vi "Testschedulev2.vi"() -> ()   [LabVIEW 2014]
uses:
  <vilib>/Utility/miscctls.llb/LVRowAndColumnTypeDef.ctl
  <vilib>/Utility/miscctls.llb/LVBoundsTypeDef.ctl
  <vilib>/event_ctls.llb/eventvkey.ctl
  <vilib>/platform/TimedLoop/XDataNode/XDataNode.xnode
  <vilib>/Platform/TimedLoop/XDataNode/timing_clust.ctl
  <vilib>/Platform/TimedLoop/XDataNode/XDNodeRunTimeDep.lvlib
  <vilib>/Platform/TimedLoop/XDataNode/wakeup.ctl
  <vilib>/Platform/TimedLoop/XDataNode/nitl_modes.ctl
panel:
  in  "Loop Number":i32
  in  "Test Flow rate g/s":i32
  in  "Test Type":u16(ring) items=["CO Lightoff", "HC Lightoff", "NO Lightoff", "OSC", "Ageing", "Leak"]
  out "Test Start":bool
  out "Loop Number":i32
  in  "Test Ready":bool
  in  "% Complete":i32(slide) scale=0.0..100.0
  in  "Time to Complete":dbl
  in  "Main TC":i32
  in  "Fan Speed V":i32
  in  "Inlet Temperature (°C)":i32
  in  "Cycle Name":string
  in  "Cycle Length":i32
  in  "Test Number":i32
  in  "Test Type Items":string[](array[string])=["CO Lightoff", "HC Lightoff", "NO Lightoff", "OSC", "Ageing", "Leak"]
  in  "TC Items":string[](array[string])=["TC1", "TC2", "TC3", "TC4", "TC5", "TC6"]
  in  "Recipe Items":string[](array[string])=["LeanspikeV1.eyes", "RAT060619Z1.eyes", "RAT181206KTM617.eyes", "RAT181217RichSpike.eyes", "RAT190207KTM934.eyes", "RAT190319KTM943Tune.eyes", "RAT190401.eyes", "RAT190405.eyes", "RAT190405e.eyes", "RAT190405f.eyes", "RAT190405g.eyes", "RAT190405h.eyes", "RAT190405i.eyes", "RAT190405j.eyes", "RAT190405k.eyes", "RAT190405L.eyes", "RAT190405M.eyes", "RAT190405N.eyes", "RAT190405O.eyes", "RAT190405P.eyes", "RAT190405Q.eyes", "RAT190405R.eyes", "RAT190405S.eyes", "RAT190405T.eyes", "RAT190405U.eyes", "RAT190405V.eyes", "RAT190405W.eyes", "RAT190405Y.eyes", "RAT190405Y2.eyes", "RAT190405Z.eyes", "RATAMP.eyes", "Richspike.eyes", "ZERO.eyes"]
  in  "Test Size":i32=2
  in  "Selection Finished":bool
  in  "Duration":i32=10 min=0
  in  "Recipe":u16(ring)=32 items=["LeanspikeV1.eyes", "RAT060619Z1.eyes", "RAT181206KTM617.eyes", "RAT181217RichSpike.eyes", "RAT190207KTM934.eyes", "RAT190319KTM943Tune.eyes", "RAT190401.eyes", "RAT190405.eyes", "RAT190405e.eyes", "RAT190405f.eyes", "RAT190405g.eyes", "RAT190405h.eyes", "RAT190405i.eyes", "RAT190405j.eyes", "RAT190405k.eyes", "RAT190405L.eyes", "RAT190405M.eyes", "RAT190405N.eyes", "RAT190405O.eyes", "RAT190405P.eyes", "RAT190405Q.eyes", "RAT190405R.eyes", "RAT190405S.eyes", "RAT190405T.eyes", "RAT190405U.eyes", "RAT190405V.eyes", "RAT190405W.eyes", "RAT190405Y.eyes", "RAT190405Y2.eyes", "RAT190405Z.eyes", "RATAMP.eyes", "Richspike.eyes", "ZERO.eyes"]
  in  "TC":u16(ring) items=["TC1", "TC2", "TC3", "TC4", "TC5", "TC6"]
  in  "Temperature":i32=10 min=0
  in  "Flow":i32=10 min=0
  out "Test Schedule":string[][](table)=[["OSC", "0", "ZERO.eyes", "0", "0", "TC1"], ["OSC", "0", "ZERO.eyes", "0", "0", "TC1"]]
  in  "Update Recipe List":bool
  out "Listbox":i32(listbox)
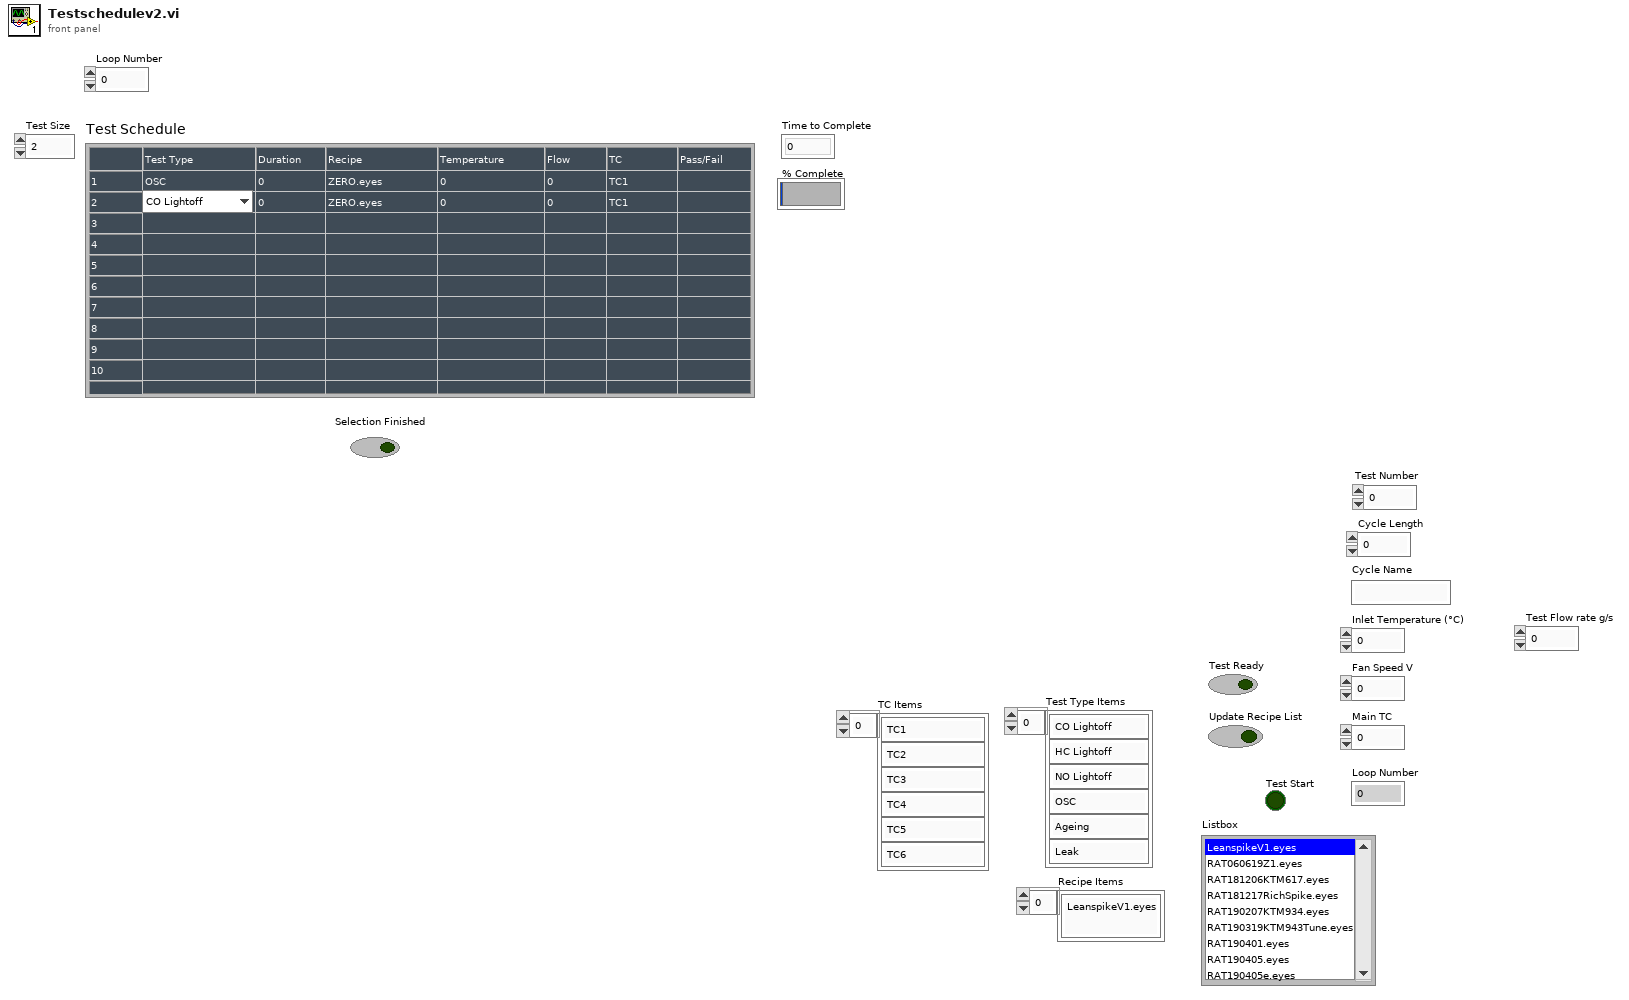
[diagram p1: front panel]
types:
  T1 = cluster{"Test Type":u16, "Duration":i32, "Recipe":u16, "Temperature":i32, "Flow":i32, "TC":u16}
  T2 = typedef "LVRowAndColumnTypeDef.ctl" = cluster{"Row":i32, "Column":i32}
  T3 = cluster{"Test Type":u16, "Duration":i32, "Recipe":u16, "Temperature":i32, "Flow":i32, "TC":u16}[]
  T4 = cluster{i32[], i32[], "Recipe":string[], i32[], i32[], i32[], bool[]}
  T5 = typedef "LVBoundsTypeDef.ctl" = cluster{"Width":u32, "Height":u32}
  T6 = typedef "eventvkey.ctl" = enum16{"ASCII", "Enter", "Return", "Shift", "Ctrl", "Alt", "Cmd", "Opt", "Caps", "NumLock", "Clear", "Break", "Up", "Down", "Left", "Right", "Insert", "Delete", "Home", "End", "PageUp", "PageDown", "Escape", "Help", "Pause", "ScrollLock", "F1", "F2", "F3", "F4", "F5", "F6", "F7", "F8", "F9", "F10", "F11", "F12", "F13", "F14", "F15", "F16", "F17", "F18", "F19", "F20", "F21", "F22", "F23", "F24", "Play", "VolumeUp", "VolumeDown", "Mute", "Two Byte Char"}
  T7 = typedef "LVPoint32TypeDef.ctl" = cluster{"Horizontal":i32, "Vertical":i32}
  T8 = typedef "LVPositionTypeDef.ctl" = cluster{"Left":i32, "Top":i32}
  T9 = cluster{"Shift":bool, "Ctrl":bool, "Alt":bool, "Cmd":bool, "Opt":bool}
  T10 = cluster{"Array":string[], "Array 2":string[], "Array 3":string[], "Array 4":string[], "Array 5":string[], "Array 6":string[]}
  T11 = cluster{i32[], i32[], "Array 3":string[], i32[], i32[], i32[], bool[]}
  T12 = cluster{i32, i32, "Combo Box":string, i32, i32, "index":i32}
  T13 = typedef "XDNodeRunTimeDep.lvlib/timing_clust.ctl" = cluster{"Expected End [f-1]":u64, "Actual End [f-1]":u64, "Finished Late? [f-1]":bool, "Expected End [i-1]":u64, "Actual End [i-1]":u64, "Finished Late? [i-1]":bool, "Expected Start [i]":u64, "Actual Start [i]":u64, "Expected Start [f]":u64, "Actual Start [f]":u64, "Source Name":string, "Structure Name":string, "Period":i64, "Deadline":i64, "Offset":i64, "Start":i64, "Priority":i32, "Timeout":i32, "Mode":T14, "Wakeup Reason":T15, "Error":errorcluster, "Source Type":string, "Secondary Source Type":string, "Global End Time":u64, "Global Start Time":u64, "Frame Duration":u64, "Iteration Duration":u64, "Assigned CPU":i32, "I/O Scan Engine Mode":u32}
  T14 = typedef "XDNodeRunTimeDep.lvlib/nitl_modes.ctl" = enum32{"No Change", "Process missed periods, maintain original phase", "Discard missed periods, maintain original phase", "Process missed periods, ignore original phase", "Discard missed periods, ignore original phase"}
  T15 = typedef "XDNodeRunTimeDep.lvlib/wakeup.ctl" = enum32{"Normal", "Aborted", "Asynchronous wakeup", "Timing source error", "Timed loop error", "Timeout"}
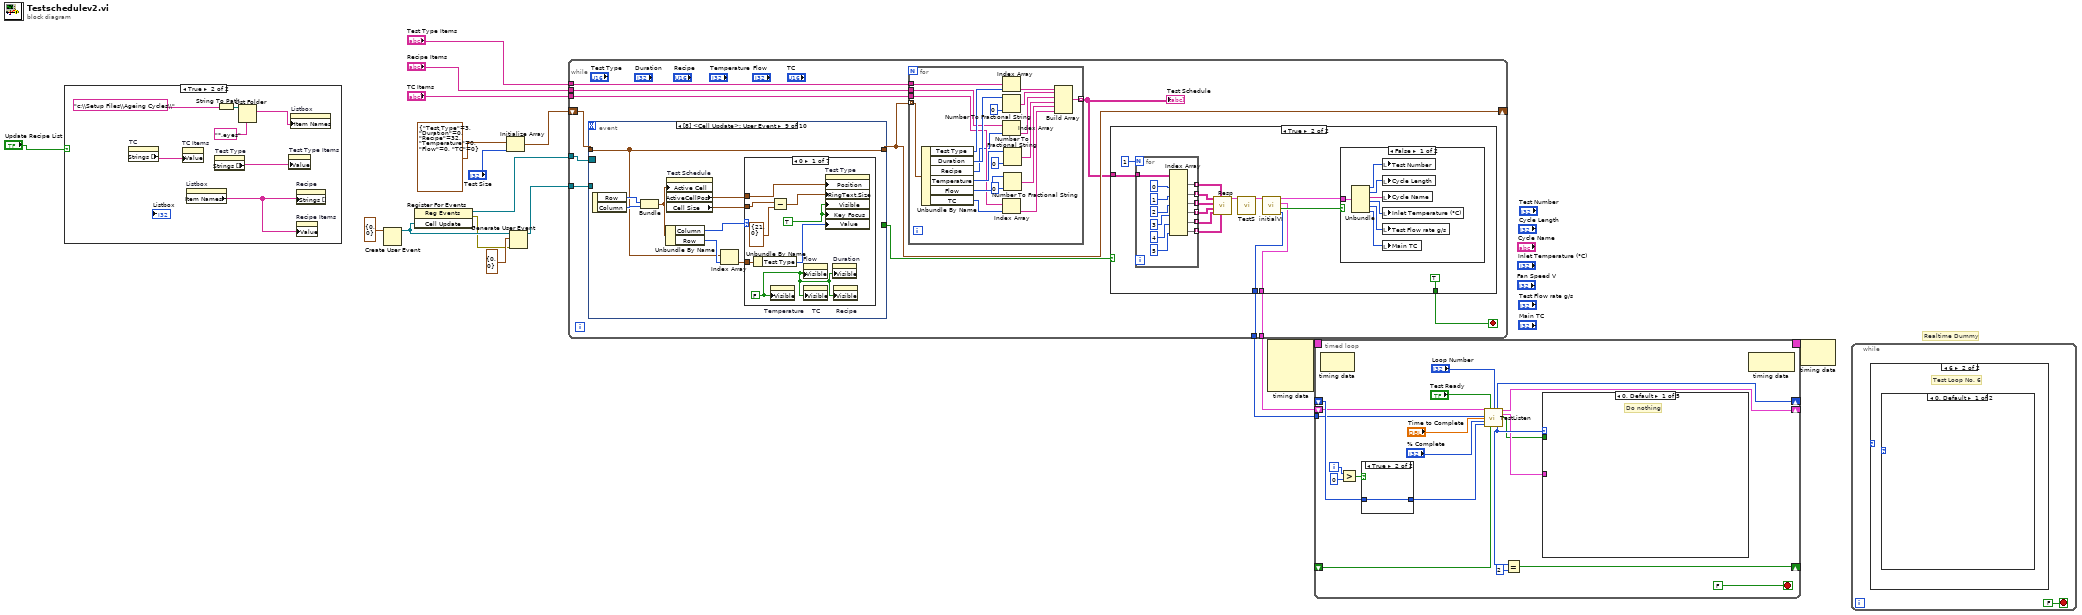
[diagram p0: block diagram]
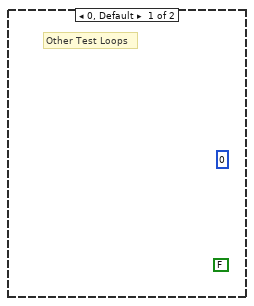
[diagram p2: hidden frame]
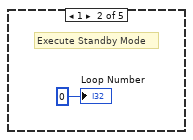
[diagram p4: hidden frame]
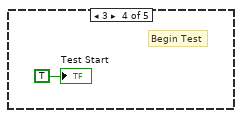
[diagram p6: hidden frame]
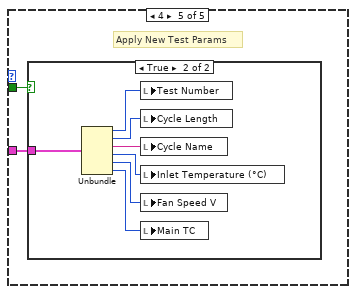
[diagram p7: hidden frame]
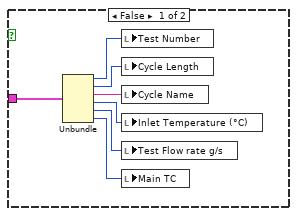
[diagram p8: hidden frame]
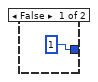
[diagram p9: hidden frame]
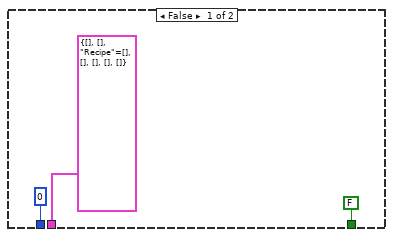
[diagram p10: hidden frame]
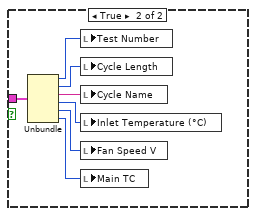
[diagram p11: hidden frame]
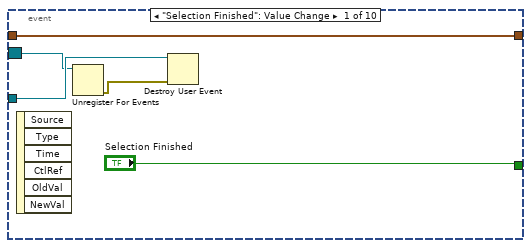
[diagram p12: hidden frame]
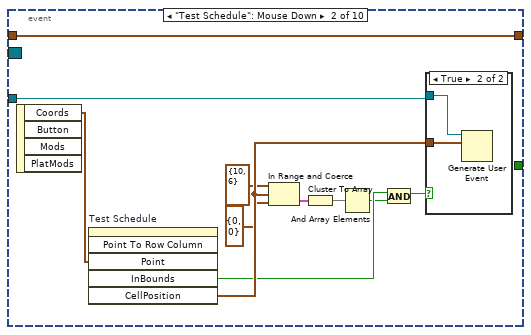
[diagram p13: hidden frame]
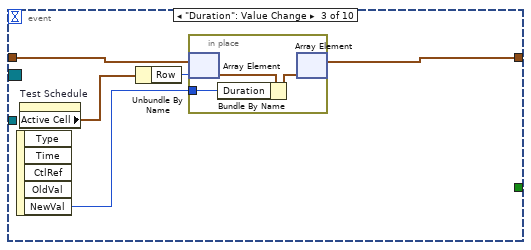
[diagram p15: hidden frame]
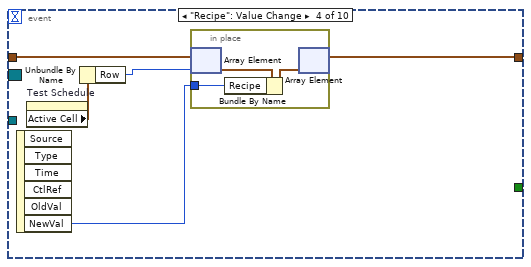
[diagram p16: hidden frame]
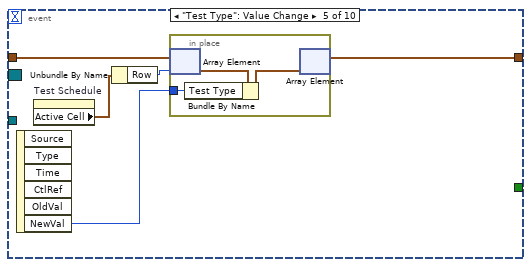
[diagram p17: hidden frame]
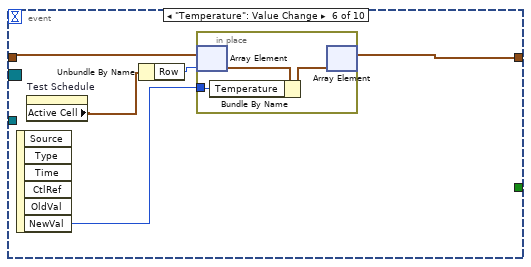
[diagram p18: hidden frame]
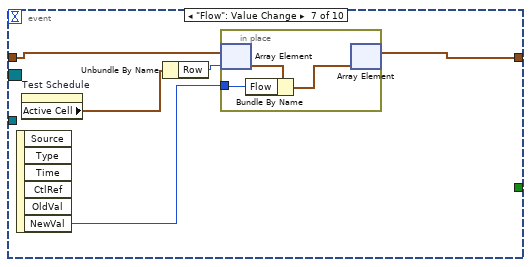
[diagram p19: hidden frame]
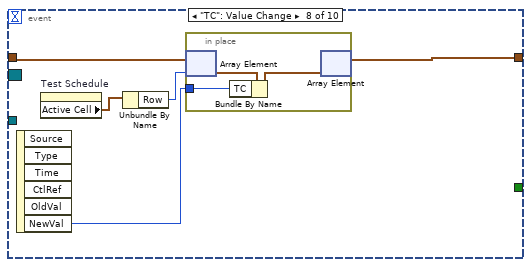
[diagram p20: hidden frame]
diagram:
  # "Realtime Dummy"
  n1 = case shown="True" "Update Recipe List" {
    frame False {
    }
    frame True {
      n2 = property on="TC" class="Ring (strict)"() -> ("Strings []"=w20:string[])  [unwired: 2 in, 2 out]
      n3 = property on="TC Items" class="Arr (strict)"("Value"=w20) -> ()  [unwired: 2 in, 2 out]
      n4 = property on="Listbox" class="LstBox (strict)"() -> ("Item Names"=w19:string[])  [unwired: 2 in, 2 out]
      n5 = property on="Test Type" class="Ring (strict)"() -> ("Strings []"=w18:string[])  [unwired: 2 in, 2 out]
      n6 = String To Path(string="c:\\Setup Files\\Ageing Cycles\\") -> (path=w24:path)
      n7 = List Folder(path=w24, pattern="*.eyes") -> (filenames=w21:string[])  [unwired: 2 in, 3 out]
      n8 = property on="Test Type Items" class="Arr (strict)"("Value"=w18) -> ()  [unwired: 2 in, 2 out]
      n9 = property on="Listbox" class="LstBox (strict)"("Item Names"=w21) -> ()  [unwired: 2 in, 2 out]
      n10 = property on="Recipe" class="Ring (strict)"("Strings []"=w19) -> ()  [unwired: 2 in, 2 out]
      n11 = property on="Recipe Items" class="Arr (strict)"("Value"=w19) -> ()  [unwired: 2 in, 2 out]
    }
  }
  n12 = Create User Event(user event datatype=T2 {"Row"=0, "Column"=0} ("Cell Update")) -> (user event=w11:refnum<user-event>)  [unwired: 1 in, 1 out]
  n13 = register-events(w11) -> (reference out=w13:refnum<event-registration>, error out=w9:errorcluster)  [unwired: 2 in]
  n14 = Initialize Array(T1 {"Test Type"=3, "Duration"=0, "Recipe"=32, "Temperature"=0, "Flow"=0, "TC"=0} ("Dilution Product Selection"), "Test Size") -> (w15:T3)
  n15 = Generate User Event(user event=w11, event data cluster=T2 {"Row"=0, "Column"=0} ("event data"), error in=w9) -> (user event out=w8:refnum<user-event>)  [unwired: 1 in, 1 out]
  n16 = while {
    shift-right: [w34] -> _
    shift-left: w15 -> [w36]
    tunnel: w13 -> [w35]
    tunnel: w8 -> [w33]
    tunnel: "Test Type Items" -> [w32]
    tunnel: "Recipe Items" -> [w31]
    tunnel: "TC Items" -> [w30]
    tunnel: [w28] -> w2
    tunnel: [w27] -> w1
    stop <- w26 stop-if-true
    n17 = event shown="[8] <Cell Update>: User Event" {
      selector: w35 -> [w104 _ _ _ _ _ _ _ _ _]
      dyn-events: _ -> [_ _ _ _ _ _ _ _ _ _]
      timeout: _ -> [_ _ _ _ _ _ _ _ _ _]
      tunnel: w36 -> [w106 w109 w124 w131 w140 w145 w154 w162 w168 w241]
      tunnel: [w106 w109 w122 w128 w138 w144 w152 w160 w168 w241] -> w34
      tunnel: w33 -> [w105 w108 _ _ _ _ _ _ _ w219]
      tunnel: ["Selection Finished" _ _ _ _ _ _ _ _ _] -> w25
      event "Selection Finished": Value Change {
        n18 = event-data() -> ()  [unwired: 1 in, 6 out]
        n19 = Destroy User Event(user event=w105) -> (error out=w103:errorcluster)  [unwired: 1 in]
        n20 = Unregister For Events(event registration refnum=w104, error in=w103) -> ()  [unwired: 1 out]
      }
      event "Test Schedule": Mouse Down {
        n21 = event-data() -> ("Coords"=w107:T7)  [unwired: 1 in, 3 out]
        n22 = invoke on="Test Schedule" class="Tbl (strict)" method="Point To Row Column"("Point"=w107) -> ("InBounds"=w113:bool, "CellPosition"=w117:T2)  [unwired: 5 in, 4 out]
        n23 = In Range and Coerce(upper limit=T2 {"Row"=10, "Column"=6}, x=w117, lower limit=T2 {"Row"=0, "Column"=0}) -> (In Range?=w114:cluster{"Row":bool, "Column":bool})  [unwired: 1 out]
        n24 = Cluster To Array(cluster=w114) -> (array=w111:bool[])
        n25 = And Array Elements(Boolean array=w111) -> (logical AND=w110:bool)
        n26 = And(x=w113, y=w110) -> (x .and. y?=w112:bool)
        n27 = case shown="True" w112 {
          tunnel: w117 -> [_ w119]
          tunnel: w108 -> [_ w118]
          frame False {
          }
          frame True {
            n28 = Generate User Event(user event=w118, event data cluster=w119) -> ()  [unwired: 2 in, 2 out]
          }
        }
      }
      event "Duration": Value Change {
        n29 = event-data() -> ("NewVal"=w121:i32)  [unwired: 1 in, 4 out]
        n30 = property on="Test Schedule" class="Tbl (strict)"() -> ("Active Cell"=w120:T2)  [unwired: 2 in, 2 out]
        n31 = Unbundle By Name(w120) -> ("Row"=w123:i32)
        n32 = in-place {
          in-place-border: w121 -> [w125]
          n33 = in-place-array #1(w124, w123) -> (w127:T1)
          n34 = Bundle By Name(cluster=w127, "Duration"=w125) -> (w126:T1)
          n35 = in-place-array #1(w126) -> (w122:T3)  [unwired: 1 out]
        }
      }
      event "Recipe": Value Change {
        n36 = event-data() -> ("NewVal"=w129:u16)  [unwired: 1 in, 5 out]
        n37 = property on="Test Schedule" class="Tbl (strict)"() -> ("Active Cell"=w132:T2)  [unwired: 2 in, 2 out]
        n38 = Unbundle By Name(w132) -> ("Row"=w130:i32)
        n39 = in-place {
          in-place-border: w129 -> [w133]
          n40 = in-place-array #2(w131, w130) -> (w135:T1)
          n41 = Bundle By Name(cluster=w135, "Recipe"=w133) -> (w134:T1)
          n42 = in-place-array #2(w134) -> (w128:T3)  [unwired: 1 out]
        }
      }
      event "Test Type": Value Change {
        n43 = event-data() -> ("NewVal"=w136:u16)  [unwired: 1 in, 5 out]
        n44 = property on="Test Schedule" class="Tbl (strict)"() -> ("Active Cell"=w137:T2)  [unwired: 2 in, 2 out]
        n45 = Unbundle By Name(w137) -> ("Row"=w139:i32)
        n46 = in-place {
          in-place-border: w136 -> [w141]
          n47 = in-place-array #3(w140, w139) -> (w143:T1)
          n48 = Bundle By Name(cluster=w143, "Test Type"=w141) -> (w142:T1)
          n49 = in-place-array #3(w142) -> (w138:T3)  [unwired: 1 out]
        }
      }
      event "Temperature": Value Change {
        n50 = event-data() -> ("NewVal"=w147:i32)  [unwired: 1 in, 5 out]
        n51 = property on="Test Schedule" class="Tbl (strict)"() -> ("Active Cell"=w146:T2)  [unwired: 2 in, 2 out]
        n52 = Unbundle By Name(w146) -> ("Row"=w148:i32)
        n53 = in-place {
          in-place-border: w147 -> [w149]
          n54 = in-place-array #4(w145, w148) -> (w151:T1)
          n55 = Bundle By Name(cluster=w151, "Temperature"=w149) -> (w150:T1)
          n56 = in-place-array #4(w150) -> (w144:T3)  [unwired: 1 out]
        }
      }
      event "Flow": Value Change {
        n57 = event-data() -> ("NewVal"=w153:i32)  [unwired: 1 in, 5 out]
        n58 = property on="Test Schedule" class="Tbl (strict)"() -> ("Active Cell"=w155:T2)  [unwired: 2 in, 2 out]
        n59 = Unbundle By Name(w155) -> ("Row"=w156:i32)
        n60 = in-place {
          in-place-border: w153 -> [w157]
          n61 = in-place-array #5(w154, w156) -> (w159:T1)
          n62 = Bundle By Name(cluster=w159, "Flow"=w157) -> (w158:T1)
          n63 = in-place-array #5(w158) -> (w152:T3)  [unwired: 1 out]
        }
      }
      event "TC": Value Change {
        n64 = event-data() -> ("NewVal"=w161:u16)  [unwired: 1 in, 5 out]
        n65 = property on="Test Schedule" class="Tbl (strict)"() -> ("Active Cell"=w164:T2)  [unwired: 2 in, 2 out]
        n66 = Unbundle By Name(w164) -> ("Row"=w163:i32)
        n67 = in-place {
          in-place-border: w161 -> [w165]
          n68 = in-place-array #6(w162, w163) -> (w167:T1)
          n69 = Bundle By Name(cluster=w167, "TC"=w165) -> (w166:T1)
          n70 = in-place-array #6(w166) -> (w160:T3)  [unwired: 1 out]
        }
      }
      event User Event {
        n71 = event-data() -> ("Row"=w176:i32, "Column"=w175:i32)  [unwired: 1 in]
        n72 = Bundle("Row"=w176, "Column"=w175) -> (w171:cluster{"Row":i32, "Column":i32})  [unwired: 1 in]
        n73 = Unbundle By Name(w171) -> ("Column"=w172:i32, "Row"=w170:i32)
        n74 = property on="Test Schedule" class="Tbl (strict)"("Active Cell"=w171) -> ("ActiveCellPos"=w174:T8, "Cell Size"=w173:T5)  [unwired: 2 in, 2 out]
        n75 = Index Array(array=w168, index=w170) -> (element=w169:T1)
        n76 = case shown="0" w172 {
          tunnel: w174 -> [w180 w190 w194 w203 w209 w217 _]
          tunnel: w173 -> [w183 w189 w198 w202 w208 w216 _]
          tunnel: w169 -> [w182 w188 w196 w204 w210 w214 _]
          frame 0 {
            w181 = FALSE ("Visible")
            w178 = TRUE ("Key Focus")
            n77 = Unbundle By Name(w182) -> ("Test Type"=w177:u16)
            n78 = property on="Temperature" class="DigNum (strict)"("Visible"=w181) -> ()  [unwired: 2 in, 2 out]
            n79 = Subtract(x=w183, y=T5 {"Width"=21, "Height"=0} ("x")) -> (x-y=w179:T5)
            n80 = property on="Flow" class="DigNum (strict)"("Visible"=w181) -> ()  [unwired: 2 in, 2 out]
            n81 = property on="TC" class="Ring (strict)"("Visible"=w181) -> ()  [unwired: 2 in, 2 out]
            n82 = property on="Test Type" class="Ring (strict)"("Position"=w180, "RingText.Size"=w179, "Visible"=w178, "Key Focus"=w178, "Value"=w177) -> ()  [unwired: 2 in, 2 out]
            n83 = property on="Duration" class="DigNum (strict)"("Visible"=w181) -> ()  [unwired: 2 in, 2 out]
            n84 = property on="Recipe" class="Ring (strict)"("Visible"=w181) -> ()  [unwired: 2 in, 2 out]
          }
          frame 1 {
            w187 = FALSE ("Visible")
            w186 = TRUE ("Key Focus")
            n85 = Unbundle By Name(w188) -> ("Duration"=w185:i32)
            n86 = property on="Temperature" class="DigNum (strict)"("Visible"=w187) -> ()  [unwired: 2 in, 2 out]
            n87 = property on="Duration" class="DigNum (strict)"("Position"=w190, "NumText.Size"=w189, "Visible"=w186, "Key Focus"=w186, "Value"=w185) -> ()  [unwired: 2 in, 2 out]
            n88 = property on="Flow" class="DigNum (strict)"("Visible"=w187) -> ()  [unwired: 2 in, 2 out]
            n89 = property on="TC" class="Ring (strict)"("Visible"=w187) -> ()  [unwired: 2 in, 2 out]
            n90 = property on="Recipe" class="Ring (strict)"("Visible"=w187) -> ()  [unwired: 2 in, 2 out]
            n91 = property on="Test Type" class="Ring (strict)"("Visible"=w187) -> ()  [unwired: 2 in, 2 out]
          }
          frame 2 {
            w193 = FALSE ("Visible")
            w192 = TRUE ("Key Focus")
            n92 = Unbundle By Name(w196) -> ("Recipe"=w191:u16)
            n93 = property on="Temperature" class="DigNum (strict)"("Visible"=w193) -> ()  [unwired: 2 in, 2 out]
            n94 = Subtract(x=w198, y=T5 {"Width"=21, "Height"=0} ("x")) -> (x-y=w195:T5)
            n95 = property on="Recipe" class="Ring (strict)"("Position"=w194, "RingText.Size"=w195, "Visible"=w192, "Key Focus"=w192, "Value"=w191) -> ()  [unwired: 2 in, 2 out]
            n96 = property on="Flow" class="DigNum (strict)"("Visible"=w193) -> ()  [unwired: 2 in, 2 out]
            n97 = property on="TC" class="Ring (strict)"("Visible"=w193) -> ()  [unwired: 2 in, 2 out]
            n98 = property on="Duration" class="DigNum (strict)"("Visible"=w193) -> ()  [unwired: 2 in, 2 out]
            n99 = property on="Test Type" class="Ring (strict)"("Visible"=w193) -> ()  [unwired: 2 in, 2 out]
          }
          frame 3 {
            w201 = FALSE
            w200 = TRUE ("Key Focus")
            n100 = Unbundle By Name(w204) -> ("Temperature"=w199:i32)
            n101 = property on="TC" class="Ring (strict)"("Visible"=w201) -> ()  [unwired: 2 in, 2 out]
            n102 = property on="Recipe" class="Ring (strict)"("Visible"=w201) -> ()  [unwired: 2 in, 2 out]
            n103 = property on="Flow" class="DigNum (strict)"("Visible"=w201) -> ()  [unwired: 2 in, 2 out]
            n104 = property on="Temperature" class="DigNum (strict)"("Position"=w203, "NumText.Size"=w202, "Visible"=w200, "Key Focus"=w200, "Value"=w199) -> ()  [unwired: 2 in, 2 out]
            n105 = property on="Duration" class="DigNum (strict)"("Visible"=w201) -> ()  [unwired: 2 in, 2 out]
            n106 = property on="Test Type" class="Ring (strict)"("Visible"=w201) -> ()  [unwired: 2 in, 2 out]
          }
          frame 4 {
            w207 = FALSE
            w206 = TRUE ("Key Focus")
            n107 = Unbundle By Name(w210) -> ("Flow"=w205:i32)
            n108 = property on="TC" class="Ring (strict)"("Visible"=w207) -> ()  [unwired: 2 in, 2 out]
            n109 = property on="Temperature" class="DigNum (strict)"("Visible"=w207) -> ()  [unwired: 2 in, 2 out]
            n110 = property on="Duration" class="DigNum (strict)"("Visible"=w207) -> ()  [unwired: 2 in, 2 out]
            n111 = property on="Flow" class="DigNum (strict)"("Position"=w209, "NumText.Size"=w208, "Visible"=w206, "Key Focus"=w206, "Value"=w205) -> ()  [unwired: 2 in, 2 out]
            n112 = property on="Test Type" class="Ring (strict)"("Visible"=w207) -> ()  [unwired: 2 in, 2 out]
            n113 = property on="Recipe" class="Ring (strict)"("Visible"=w207) -> ()  [unwired: 2 in, 2 out]
          }
          frame 5 {
            w213 = FALSE
            w212 = TRUE ("Key Focus")
            n114 = Unbundle By Name(w214) -> ("TC"=w211:u16)
            n115 = property on="Temperature" class="DigNum (strict)"("Visible"=w213) -> ()  [unwired: 2 in, 2 out]
            n116 = Subtract(x=w216, y=T5 {"Width"=21, "Height"=0} ("x")) -> (x-y=w215:T5)
            n117 = property on="TC" class="Ring (strict)"("Position"=w217, "RingText.Size"=w215, "Visible"=w212, "Key Focus"=w212, "Value"=w211) -> ()  [unwired: 2 in, 2 out]
            n118 = property on="Duration" class="DigNum (strict)"("Visible"=w213) -> ()  [unwired: 2 in, 2 out]
            n119 = property on="Flow" class="DigNum (strict)"("Visible"=w213) -> ()  [unwired: 2 in, 2 out]
            n120 = property on="Test Type" class="Ring (strict)"("Visible"=w213) -> ()  [unwired: 2 in, 2 out]
            n121 = property on="Recipe" class="Ring (strict)"("Visible"=w213) -> ()  [unwired: 2 in, 2 out]
          }
          frame Default {
          }
        }
      }
      event "Duration": Key Down? {
        n122 = event-data() -> ("PlatMods"=w220:T9, "Char"=w228:i16, "VKey"=w224:T6)  [unwired: 1 in]
        n123 = property on="Test Schedule" class="Tbl (strict)"() -> ("Active Cell"=w234:T2)  [unwired: 2 in, 2 out]
        n124 = Unbundle By Name(w234) -> ("Row"=w239:i32, "Column"=w240:i32)
        n125 = Unbundle By Name(w220) -> ("Shift"=w235:bool)
        n126 = case shown="True" w235 {
          tunnel: w240 -> [w252 w261]
          tunnel: w239 -> [w248 w257]
          tunnel: [w245 w254] -> w238
          tunnel: [w244 w253] -> w237
          frame False {
            n127 = Increment(x=w252) -> (x+1=w251:i32)
            n128 = Quotient & Remainder(x=w251, y=3) -> (x-y*floor(x/y)=w244:i32, floor(x/y)=w249:i32)
            n129 = Add(x=w248, y=w249) -> (x+y=w247:i32)
            n130 = Quotient & Remainder(x=w247, y=10) -> (x-y*floor(x/y)=w245:i32)  [unwired: 1 out]
          }
          frame True {
            n131 = Decrement(x=w261) -> (x-1=w260:i32)
            n132 = Quotient & Remainder(x=w260, y=3) -> (x-y*floor(x/y)=w253:i32, floor(x/y)=w258:i32)
            n133 = Add(x=w257, y=w258) -> (x+y=w256:i32)
            n134 = Quotient & Remainder(x=w256, y=10) -> (x-y*floor(x/y)=w254:i32)  [unwired: 1 out]
          }
        }
        n135 = Concatenate Strings("\t") -> (w232:string)
        n136 = Build Array(eventvkey."Enter" ("VKey"), eventvkey."Return" ("VKey")) -> (w225:T6[])
        n137 = String To Byte Array(string=w232) -> (unsigned byte array=w231:u8[])
        n138 = Search 1D Array(1D array=w231, element=w228) -> (index of element=w230:i32)  [unwired: 1 in]
        n139 = Search 1D Array(1D array=w225, element=w224) -> (index of element=w223:i32)  [unwired: 1 in]
        n140 = Greater Or Equal To 0?(x=w230) -> (x >= 0?=w229:bool)
        n141 = Greater Or Equal To 0?(x=w223) -> (x >= 0?=w221:bool)
        n142 = Or(x=w229, y=w221) -> (x .or. y?=w222:bool)
        n143 = Bundle(w238, w237) -> (w236:cluster{i32, i32})  [unwired: 1 in]
        n144 = case shown="True" w222 {
          tunnel: w236 -> [_ w243]
          tunnel: w219 -> [_ w242]
          frame False {
          }
          frame True {
            n145 = Generate User Event(user event=w242, event data cluster=w243) -> ()  [unwired: 2 in, 2 out]
          }
        }
        n146 = event-data("Discard?"=w222) -> ()  [unwired: 6 in, 1 out]
      }
    }
    n147 = for {
      tunnel: [w100] -> w29 mode=indexing
      tunnel: w34 -> [w99] mode=indexing
      tunnel: w32 -> [w97]
      tunnel: w31 -> [w90]
      tunnel: w30 -> [w89]
      n148 = Unbundle By Name(w99) -> ("Test Type"=w96:u16, "Duration"=w101:i32, "Recipe"=w88:u16, "Temperature"=w95:i32, "Flow"=w94:i32, "TC"=w87:u16)
      n149 = Index Array(array=w97, index=w96) -> (element=w98:string)
      n150 = Number To Fractional String(number=w101, precision (6)=i16 0) -> (F-format string=w93:string)  [unwired: 2 in]
      n151 = Index Array(array=w90, index=w88) -> (element=w86:string)
      n152 = Index Array(array=w89, index=w87) -> (element=w85:string)
      n153 = Number To Fractional String(number=w95, precision (6)=i16 0) -> (F-format string=w92:string)  [unwired: 2 in]
      n154 = Number To Fractional String(number=w94, precision (6)=i16 0) -> (F-format string=w91:string)  [unwired: 2 in]
      n155 = Build Array(w98, w93, w86, w92, w91, w85) -> (w100:string[])
    }
    "Test Schedule" <- w29
    n156 = case shown="True" w25 {
      tunnel: w29 -> [_ w54]
      tunnel: [FALSE TRUE] -> w26
      tunnel: [T4 {[], [], "Recipe"=[], [], [], [], []} ("Queue cluster") w40] -> w28
      tunnel: [0 ("Max No. of Tests") w43] -> w27
      frame False {
      }
      frame True {
        n157 = for {
          N: 1 -> [_]
          tunnel: [w75] -> w51 mode=indexing
          tunnel: [w74] -> w50 mode=indexing
          tunnel: [w73] -> w49 mode=indexing
          tunnel: [w72] -> w48 mode=indexing
          tunnel: [w71] -> w47 mode=indexing
          tunnel: [w70] -> w44 mode=indexing
          tunnel: w54 -> [w69]
          n158 = Index Array(array=w69, index (col) #1=0 ("disabled index (col)"), index (col) #2=1 ("index (col)"), index (col) #3=2 ("index (col)"), index (col) #4=3 ("index (col)"), index (col) #5=4 ("index (col)"), index (col) #6=5 ("index (col)")) -> (element #1=w75:string[], element #2=w74:string[], element #3=w73:string[], element #4=w72:string[], element #5=w71:string[], element #6=w70:string[])  [unwired: 6 in]
        }
        n159 = call "Resp.vi"("Array 6"=w44, "Array"=w51, "Array 5"=w47, "Array 4"=w48, "Array 3"=w49, "Array 2"=w50) -> ("output cluster"=w52:T10)  [unwired: 5 in]
        n160 = call "TestS.vi"("Input cluster"=w52) -> ("output cluster"=w42:T11)  [unwired: 10 in]
        n161 = call "initialVI.vi"("Input cluster"=w42) -> ("Max No. of Tests"=w43:i32, "Voltage/(g/s)"=w41:bool, "Queue cluster"=w40:T4, "Test Param"=w46:T12)  [unwired: 7 in]
        n162 = case shown="False" w41 {
          tunnel: w46 -> [w61 w68]
          frame False {
            n163 = Unbundle(w61) -> (w60:i32, w59:i32, "Combo Box"=w58:string, w57:i32, w56:i32, "index"=w55:i32)
            n164 = local write "Test Number"(w60) -> ()
            n165 = local write "Cycle Length"(w59) -> ()
            n166 = local write "Cycle Name"(w58) -> ()
            n167 = local write "Inlet Temperature (°C)"(w57) -> ()
            n168 = local write "Test Flow rate g/s"(w56) -> ()
            n169 = local write "Main TC"(w55) -> ()
          }
          frame True {
            n170 = Unbundle(w68) -> (w67:i32, w66:i32, "Combo Box"=w65:string, w64:i32, w63:i32, "index"=w62:i32)
            n171 = local write "Test Number"(w67) -> ()
            n172 = local write "Cycle Length"(w66) -> ()
            n173 = local write "Cycle Name"(w65) -> ()
            n174 = local write "Inlet Temperature (°C)"(w64) -> ()
            n175 = local write "Fan Speed V"(w63) -> ()
            n176 = local write "Main TC"(w62) -> ()
          }
        }
      }
    }
  }
  n177 = node-c288 ("Input Node")() -> (w4:T13)  [unwired: 4 in]
  n178 = timed-loop {
    shift-right: [w271] -> _
    shift-left: w2 -> [w273]
    shift-right: [w272] -> _
    shift-left: _ -> [w280]
    shift-right: [w274] -> _
    shift-left: _ -> [w269]
    timing: w4 -> [_]
    timing-out: [_] -> w3
    tunnel: w1 -> [w266]
    i -> [w276]
    stop <- FALSE stop-if-true
    n179 = node-c288() -> ()  [unwired: 1 in, 1 out]
    n180 = Greater?(x=w276, y=0) -> (0:w278:bool)
    n181 = case shown="True" w278 {
      tunnel: w280 -> [_ w303]
      tunnel: [1 ("No. of Test") w303] -> w264
      frame False {
      }
      frame True {
      }
    }
    n182 = call "TestListen.vi"("Input cluster"=w273, "Test Ready"="Test Ready", "Loop Number"="Loop Number", "Max No. of Tests"=w266, "Time to Complete"="Time to Complete", "% Complete"="% Complete", "No. of Test"=w264, "Test Finished"=w269) -> ("Test No."=w272:i32, "Queue cluster"=w271:T4, "Test Param"=w268:T12, "Voltage/(g/s)"=w263:bool, "State"=w270:i32)  [unwired: 3 in]
    n183 = Equal?(x=w270, y=2) -> (x = y?=w274:bool)
    n184 = case shown="0, Default" w270 {
      tunnel: w268 -> [_ _ _ _ w287]
      tunnel: w263 -> [_ _ _ _ w286]
      frame 0, Default {
        # "Do nothing"
      }
      frame 1 {
        # "Execute Standby Mode"
        "Loop Number" <- 0 ("Standby")
      }
      frame 2 {
        # "Intermediary state"
      }
      frame 3 {
        # "Begin Test"
        "Test Start" <- TRUE ("Test Start")
      }
      frame 4 {
        # "Apply New Test Params"
        n185 = case shown="True" w286 {
          tunnel: w287 -> [w294 w296]
          frame False {
            n186 = Unbundle(w294) -> (w293:i32, w292:i32, "Combo Box"=w291:string, w290:i32, w289:i32, "index"=w288:i32)
            n187 = local write "Test Number"(w293) -> ()
            n188 = local write "Cycle Length"(w292) -> ()
            n189 = local write "Cycle Name"(w291) -> ()
            n190 = local write "Inlet Temperature (°C)"(w290) -> ()
            n191 = local write "Test Flow rate g/s"(w289) -> ()
            n192 = local write "Main TC"(w288) -> ()
          }
          frame True {
            n193 = Unbundle(w296) -> (w301:i32, w300:i32, "Combo Box"=w299:string, w295:i32, w298:i32, "index"=w297:i32)
            n194 = local write "Test Number"(w301) -> ()
            n195 = local write "Cycle Length"(w300) -> ()
            n196 = local write "Cycle Name"(w299) -> ()
            n197 = local write "Inlet Temperature (°C)"(w295) -> ()
            n198 = local write "Fan Speed V"(w298) -> ()
            n199 = local write "Main TC"(w297) -> ()
          }
        }
      }
    }
    n200 = node-c288() -> ()  [unwired: 1 in, 1 out]
  }
  n201 = node-c288(w3) -> ()  [unwired: 1 out]
  n202 = while {
    stop <- FALSE stop-if-true
    n203 = case shown="6" {
      selector: _ -> [_ _]
      frame 0, Default {
        (unwired) FALSE
        (unwired) 0
        # "Other Test Loops"
      }
      frame 6 {
        # "Test Loop No. 6"
        n204 = case shown="0, Default" {
          selector: _ -> [_ _]
          frame 0, Default {
          }
          frame 1 {
          }
        }
      }
    }
  }
